vi "17-Calculate Apex.vi"(11 "vy":i32) -> (3 "y":dbl)   [LabVIEW 2019, in "17.lvlib"]
uses:
  17.lvlib
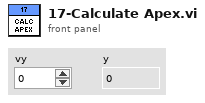
[diagram p1: front panel]
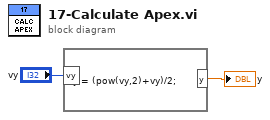
[diagram p0: block diagram]
diagram:
  n1 = formula code="y = (pow(vy,2)+vy)/2;"("vy"="vy") -> ("y"=→"y":dbl)
